vi "Finish.vi"   [LabVIEW 2023]
doc: "This VIcloses device references, sends final commands to the network tables and the joysticks, and terminates all command and control loops."
uses:
  GlobalDrivebase.vi
  GlobalDriverStationCommands.vi
  <vilib>/Rock Robotics/WPI/Utilities/WPI_GetSetVariantRefNum.vi
  GlobalMiscellaneous.vi
  GlobalElevator.vi
  GlobalNoteHandling.vi
  GlobalShooter.vi
types:
  T1 = typedef "WPI_JoystickDevRef.ctl" = cluster{"Device":T2}
  T2 = typedef "WPI_JoystickDeviceEnum.ctl" = enum16{"USB 0", "USB 1", "USB 2", "USB 3", "USB 4", "USB 5"}
  T3 = typedef "WPI_PWMDeviceRef.ctl" = cluster{"DeviceStatus":errorcluster, "PWM Channel":T4}
  T4 = typedef "FPGA_DIOPWMChannel.ctl" = enum8{"PWM 0", "PWM 1", "PWM 2", "PWM 3", "PWM 4", "PWM 5", "PWM 6", "PWM 7", "PWM 8", "PWM 9", "PWM MXP 0", "PWM MXP 1", "PWM MXP 2", "PWM MXP 3", "PWM MXP 4", "PWM MXP 5", "PWM MXP 6", "PWM MXP 7", "PWM MXP 8", "PWM MXP 9", "Invalid"}
  T5 = typedef "WPI_MotorControlDeviceRef.ctl" = cluster{"DeviceStatus":errorcluster, "Type":T6, "PWM":cluster{"PWM Channel":T4, "DeadBand":T7}, "CAN":cluster{"Device Number":u8, "SetOutput VI Ref":variant, "GetOutput VI Ref":variant, "Enable VI Ref":variant, "Disable VI Ref":variant, "Data":variant}, "Invert":bool, "DIO PWM":cluster{"PWM \"Enable\" Channel":T4, "DIOChannel":T8, "PWM Rate":dbl}}
  T6 = typedef "WPI_MotorControlType.ctl" = enum16{"PWM", "CAN", "DIO PWM"}
  T7 = typedef "WPI_PWMDeadband.ctl" = cluster{"Name":string, "maxPositivePwm":i32, "minPositivePwm":i32, "centerPwm":i32, "maxNegativePwm":i32, "minNegativePwm":i32, "angularRange":u16}
  T8 = typedef "FPGA_DIOChannel.ctl" = enum8{"DIO 0", "DIO 1", "DIO 2", "DIO 3", "DIO 4", "DIO 5", "DIO 6", "DIO 7", "DIO 8", "DIO 9", "DIO MXP 0", "DIO MXP 1", "DIO MXP 2", "DIO MXP 3", "DIO MXP 4", "DIO MXP 5", "DIO MXP 6", "DIO MXP 7", "DIO MXP 8", "DIO MXP 9", "DIO MXP 10", "DIO MXP 11", "DIO MXP 12", "DIO MXP 13", "DIO MXP 14", "DIO MXP 15", "SPI Port CS1", "SPI Port CS2", "SPI Port CS3", "SPI Port MISO", "SPI Port MOSI", "Invalid"}
  T9 = typedef "WPI_SolenoidDevRef.ctl" = cluster{"DevStatus":errorcluster, "Pneumatics Control Module":u8, "Forward Solenoid Channel":T10, "Reverse Solenoid Channel":T10}
  T10 = typedef "WPI_SolenoidChannel.ctl" = enum8{"Solenoid 0", "Solenoid 1", "Solenoid 2", "Solenoid 3", "Solenoid 4", "Solenoid 5", "Solenoid 6", "Solenoid 7", "Solenoid 8", "Solenoid 9", "Solenoid 10", "Solenoid 11", "Solenoid 12", "Solenoid 13", "Solenoid 14", "Solenoid 15", "Invalid"}
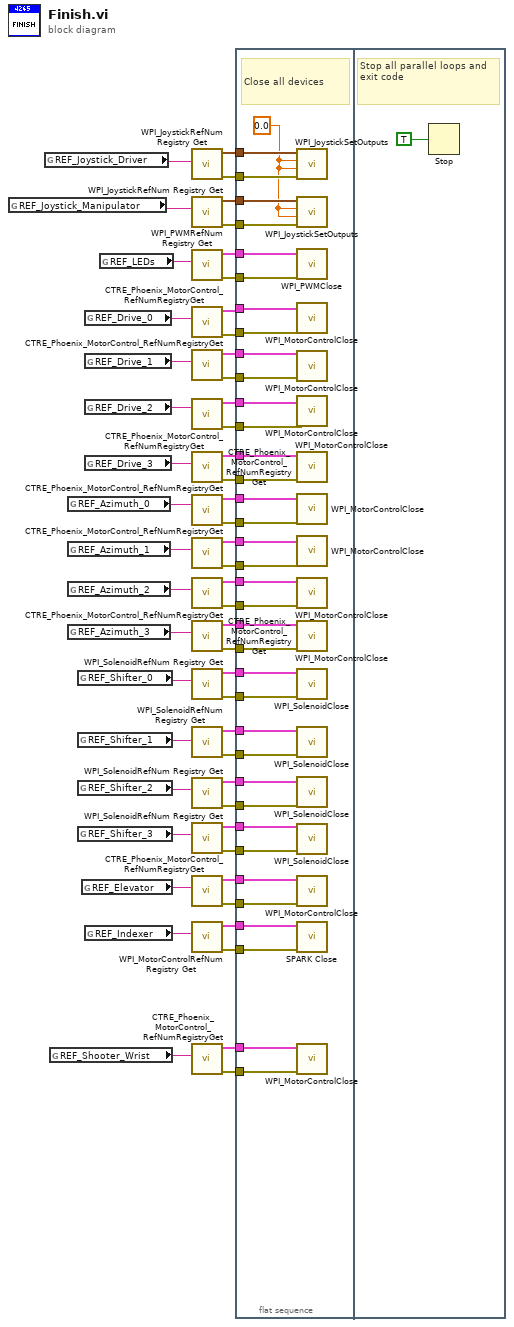
[diagram p0: block diagram]
diagram:
  n1 = global read "GlobalDriverStationCommands.vi" "REF_Joystick_Manipulator"() -> (w13:string)
  n2 = global read "GlobalDriverStationCommands.vi" "REF_Joystick_Driver"() -> (w14:string)
  n3 = global read "GlobalShooter.vi" "REF_Shooter_Wrist"() -> (w1:string)
  n4 = global read "GlobalDrivebase.vi" "REF_Azimuth_0"() -> (w26:string)
  n5 = global read "GlobalDrivebase.vi" "REF_Azimuth_1"() -> (w25:string)
  n6 = global read "GlobalDrivebase.vi" "REF_Azimuth_2"() -> (w24:string)
  n7 = global read "GlobalDrivebase.vi" "REF_Azimuth_3"() -> (w23:string)
  n8 = global read "GlobalDrivebase.vi" "REF_Shifter_0"() -> (w18:string)
  n9 = global read "GlobalDrivebase.vi" "REF_Shifter_1"() -> (w17:string)
  n10 = global read "GlobalDrivebase.vi" "REF_Shifter_2"() -> (w16:string)
  n11 = global read "GlobalDrivebase.vi" "REF_Shifter_3"() -> (w15:string)
  n12 = global read "GlobalElevator.vi" "REF_Elevator"() -> (w7:string)
  n13 = global read "GlobalDrivebase.vi" "REF_Drive_0"() -> (w22:string)
  n14 = global read "GlobalDrivebase.vi" "REF_Drive_1"() -> (w21:string)
  n15 = global read "GlobalDrivebase.vi" "REF_Drive_2"() -> (w20:string)
  n16 = global read "GlobalDrivebase.vi" "REF_Drive_3"() -> (w19:string)
  n17 = global read "GlobalNoteHandling.vi" "REF_Indexer"() -> (w4:string)
  n18 = global read "GlobalMiscellaneous.vi" "REF_LEDs"() -> (w10:string)
  n19 = call <vilib>:"WPI_JoystickRefNum Registry Get.vi"("refnum name"=w14) -> ("error out"=w53:errorcluster, "JoystickDevRef"=w54:T1)  [unwired: 9 in]
  n20 = call <vilib>:"WPI_JoystickRefNum Registry Get.vi"("refnum name"=w13) -> ("error out"=w51:errorcluster, "JoystickDevRef"=w52:T1)  [unwired: 9 in]
  n21 = call <vilib>:"WPI_PWMRefNum Registry Get.vi"("refnum name"=w10) -> ("error out"=w11:errorcluster, "PWMDeviceRef"=w12:T3)  [unwired: 9 in]
  n22 = call <vilib>:"CTRE_Phoenix_MotorControl_RefNumRegistryGet.vi"("refnum name"=w22) -> ("error out"=w45:errorcluster, "PhoenixMotorControlDevRef"=w46:T5)  [unwired: 9 in]
  n23 = call <vilib>:"CTRE_Phoenix_MotorControl_RefNumRegistryGet.vi"("refnum name"=w21) -> ("error out"=w41:errorcluster, "PhoenixMotorControlDevRef"=w44:T5)  [unwired: 9 in]
  n24 = call <vilib>:"CTRE_Phoenix_MotorControl_RefNumRegistryGet.vi"("refnum name"=w20) -> ("error out"=w42:errorcluster, "PhoenixMotorControlDevRef"=w43:T5)  [unwired: 9 in]
  n25 = call <vilib>:"CTRE_Phoenix_MotorControl_RefNumRegistryGet.vi"("refnum name"=w19) -> ("error out"=w49:errorcluster, "PhoenixMotorControlDevRef"=w50:T5)  [unwired: 9 in]
  n26 = call <vilib>:"CTRE_Phoenix_MotorControl_RefNumRegistryGet.vi"("refnum name"=w26) -> ("error out"=w36:errorcluster, "PhoenixMotorControlDevRef"=w40:T5)  [unwired: 9 in]
  n27 = call <vilib>:"CTRE_Phoenix_MotorControl_RefNumRegistryGet.vi"("refnum name"=w25) -> ("error out"=w35:errorcluster, "PhoenixMotorControlDevRef"=w39:T5)  [unwired: 9 in]
  n28 = call <vilib>:"CTRE_Phoenix_MotorControl_RefNumRegistryGet.vi"("refnum name"=w24) -> ("error out"=w34:errorcluster, "PhoenixMotorControlDevRef"=w38:T5)  [unwired: 9 in]
  n29 = call <vilib>:"CTRE_Phoenix_MotorControl_RefNumRegistryGet.vi"("refnum name"=w23) -> ("error out"=w33:errorcluster, "PhoenixMotorControlDevRef"=w37:T5)  [unwired: 9 in]
  n30 = call <vilib>:"WPI_SolenoidRefNum Registry Get.vi"("refnum name"=w18) -> ("error out"=w31:errorcluster, "SolenoidDevRef"=w32:T9)  [unwired: 9 in]
  n31 = call <vilib>:"WPI_SolenoidRefNum Registry Get.vi"("refnum name"=w17) -> ("error out"=w29:errorcluster, "SolenoidDevRef"=w30:T9)  [unwired: 9 in]
  n32 = call <vilib>:"WPI_SolenoidRefNum Registry Get.vi"("refnum name"=w16) -> ("error out"=w27:errorcluster, "SolenoidDevRef"=w28:T9)  [unwired: 9 in]
  n33 = call <vilib>:"WPI_SolenoidRefNum Registry Get.vi"("refnum name"=w15) -> ("error out"=w47:errorcluster, "SolenoidDevRef"=w48:T9)  [unwired: 9 in]
  n34 = call <vilib>:"CTRE_Phoenix_MotorControl_RefNumRegistryGet.vi"("refnum name"=w7) -> ("error out"=w8:errorcluster, "PhoenixMotorControlDevRef"=w9:T5)  [unwired: 9 in]
  n35 = call <vilib>:"WPI_MotorControlRefNum Registry Get.vi"("refnum name"=w4) -> ("error out"=w6:errorcluster, "MotorControlDevRef"=w5:T5)  [unwired: 9 in]
  n36 = call <vilib>:"CTRE_Phoenix_MotorControl_RefNumRegistryGet.vi"("refnum name"=w1) -> ("error out"=w3:errorcluster, "PhoenixMotorControlDevRef"=w2:T5)  [unwired: 9 in]
  n37 = flat-sequence {
    tunnel: w46 -> [w91]
    tunnel: w44 -> [w90]
    tunnel: w45 -> [w89]
    tunnel: w54 -> [w88]
    tunnel: w53 -> [w87]
    tunnel: w52 -> [w86]
    tunnel: w51 -> [w85]
    tunnel: w50 -> [w83]
    tunnel: w49 -> [w82]
    tunnel: w48 -> [w81]
    tunnel: w47 -> [w80]
    tunnel: w43 -> [w79]
    tunnel: w42 -> [w78]
    tunnel: w41 -> [w77]
    tunnel: w40 -> [w76]
    tunnel: w39 -> [w75]
    tunnel: w38 -> [w74]
    tunnel: w37 -> [w73]
    tunnel: w36 -> [w72]
    tunnel: w35 -> [w71]
    tunnel: w34 -> [w70]
    tunnel: w33 -> [w69]
    tunnel: w32 -> [w68]
    tunnel: w31 -> [w67]
    tunnel: w30 -> [w66]
    tunnel: w29 -> [w65]
    tunnel: w28 -> [w64]
    tunnel: w27 -> [w63]
    tunnel: w12 -> [w62]
    tunnel: w11 -> [w61]
    tunnel: w9 -> [w60]
    tunnel: w8 -> [w59]
    tunnel: w5 -> [w57]
    tunnel: w6 -> [w58]
    tunnel: w2 -> [w55]
    tunnel: w3 -> [w56]
    frame #0 {
      w84 = sgl 0.0 ("Left Rumble")
      # "Close all devices"
      n38 = call <vilib>:"WPI_JoystickSetOutputs.vi"("error in (no error)"=w87, "Right Rumble"=w84, "Left Rumble"=w84, "JoystickDevRef"=w88) -> ()  [unwired: 6 in, 2 out]
      n39 = call <vilib>:"WPI_JoystickSetOutputs.vi"("error in (no error)"=w85, "Right Rumble"=w84, "Left Rumble"=w84, "JoystickDevRef"=w86) -> ()  [unwired: 6 in, 2 out]
      n40 = call <vilib>:"WPI_PWMClose.vi"("error in (no error)"=w61, "PWMDeviceRef"=w62) -> ()  [unwired: 9 in, 1 out]
      n41 = call <vilib>:"WPI_MotorControlClose.vi"("error in"=w89, "MotorControlDevRef"=w91) -> ()  [unwired: 9 in, 1 out]
      n42 = call <vilib>:"WPI_MotorControlClose.vi"("error in"=w77, "MotorControlDevRef"=w90) -> ()  [unwired: 9 in, 1 out]
      n43 = call <vilib>:"WPI_MotorControlClose.vi"("error in"=w78, "MotorControlDevRef"=w79) -> ()  [unwired: 9 in, 1 out]
      n44 = call <vilib>:"WPI_MotorControlClose.vi"("error in"=w82, "MotorControlDevRef"=w83) -> ()  [unwired: 9 in, 1 out]
      n45 = call <vilib>:"WPI_MotorControlClose.vi"("error in"=w72, "MotorControlDevRef"=w76) -> ()  [unwired: 9 in, 1 out]
      n46 = call <vilib>:"WPI_MotorControlClose.vi"("error in"=w71, "MotorControlDevRef"=w75) -> ()  [unwired: 9 in, 1 out]
      n47 = call <vilib>:"WPI_MotorControlClose.vi"("error in"=w70, "MotorControlDevRef"=w74) -> ()  [unwired: 9 in, 1 out]
      n48 = call <vilib>:"WPI_MotorControlClose.vi"("error in"=w69, "MotorControlDevRef"=w73) -> ()  [unwired: 9 in, 1 out]
      n49 = call <vilib>:"WPI_SolenoidClose.vi"("error in (no error)"=w67, "SolenoidDevRef"=w68) -> ()  [unwired: 9 in, 1 out]
      n50 = call <vilib>:"WPI_SolenoidClose.vi"("error in (no error)"=w65, "SolenoidDevRef"=w66) -> ()  [unwired: 9 in, 1 out]
      n51 = call <vilib>:"WPI_SolenoidClose.vi"("error in (no error)"=w63, "SolenoidDevRef"=w64) -> ()  [unwired: 9 in, 1 out]
      n52 = call <vilib>:"WPI_SolenoidClose.vi"("error in (no error)"=w80, "SolenoidDevRef"=w81) -> ()  [unwired: 9 in, 1 out]
      n53 = call <vilib>:"WPI_MotorControlClose.vi"("error in"=w59, "MotorControlDevRef"=w60) -> ()  [unwired: 9 in, 1 out]
      n54 = call <vilib>:"SPARK Close.vi"("error in"=w58, "MotorControlDeviceRef"=w57) -> ()  [unwired: 9 in, 1 out]
      n55 = call <vilib>:"WPI_MotorControlClose.vi"("error in"=w56, "MotorControlDevRef"=w55) -> ()  [unwired: 9 in, 1 out]
    }
    frame #1 {
      # "Stop all parallel loops and exit code"
      n56 = Stop(stop? (T)=TRUE ("Quit")) -> ()
    }
  }
